vi "Read Capabilities.vi"(8 "error in (no error)":errorcluster, 11 "SLSC NVMEM Session In":refnum<class "SLSC Interface.lvclass">) -> (0 "error out":errorcluster, 2 "capabilities":string, 3 "SLSC NVMEM Session Out":refnum<class "SLSC Interface.lvclass">)   [LabVIEW 2015, in "SLSC Switch.lvlib" / "SLSC Switch.lvclass"]
uses:
  SLSC Switch.lvclass
  <vilib>/National Instruments/SLSC Local or Remote Interface/SLSC Interface Class/SLSC Interface.lvclass
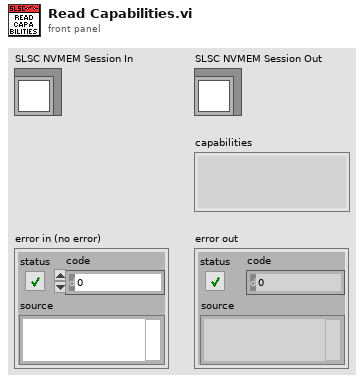
[diagram p1: front panel]
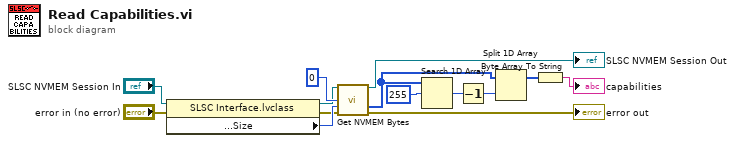
[diagram p0: block diagram]
diagram:
  n1 = property class="SLSC Interface.lvclass"(reference="SLSC NVMEM Session In", error in="error in (no error)") -> (reference out=w10:refnum<class "SLSC Interface.lvclass">, error out=w9:errorcluster, "API:session property node:NVMEM Area:NVMEMArea.Size"=w12:u32)
  n2 = call-dynamic "Get NVMEM Bytes.vi"("SLSC Interface In"=w10, "data address"=u32 0, "data size"=w12, "error in (no error)"=w9) -> ("SLSC Interface Out"=→"SLSC NVMEM Session Out":refnum<class "SLSC Interface.lvclass">, "data out"=w7:u8[], "error out"=→"error out":errorcluster)  [unwired: 7 in, 2 out]
  n3 = Search 1D Array(1D array=w7, element=u8 255) -> (index of element=w5:i32)  [unwired: 1 in]
  n4 = Decrement(x=w5) -> (x-1=w4:i32)
  n5 = Split 1D Array(array=w7, index=w4) -> (first subarray=w6:u8[])  [unwired: 1 out]
  n6 = Byte Array To String(unsigned byte array=w6) -> (string=→"capabilities":string)
